vi "OAT Demodulation with Decimation.vi"   [LabVIEW 2017, in "SoundVib_Resampling.lvlib"]
uses:
  <vilib>/addons/Sound and Vibration/Order Analysis/Resample Order Tracking/SoundVib_Resampling.lvlib
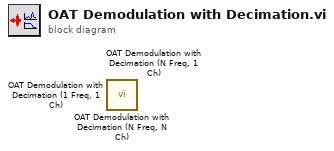
[diagram p0: block diagram]
diagram:
  n1 = call <vilib>:"OAT Demodulation with Decimation (N Freq, N Ch).vi"() -> ()  [unwired: 11 in, 5 out]
  n2 = call <vilib>:"OAT Demodulation with Decimation (N Freq, 1 Ch).vi"() -> ()  [unwired: 11 in, 5 out]
  n3 = call <vilib>:"OAT Demodulation with Decimation (1 Freq, 1 Ch).vi"() -> ()  [unwired: 12 in, 4 out]
